vi "Example Graph.vi"() -> ()   [LabVIEW 2013]
uses:
  C:/tf/play/labview/Tinkerforge.dll
  Tinkerforge.dll
panel:
  in  "stop":bool
  out "graph":i32[](graph)
  in  "uid":string="amb"
  in  "port":i32=4223
  in  "host":string="localhost"
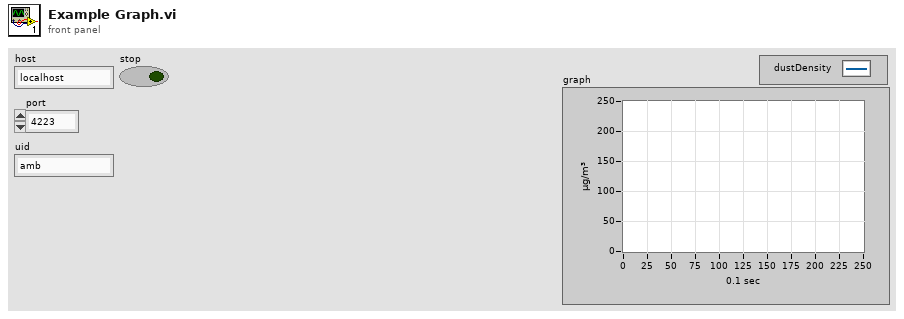
[diagram p1: front panel]
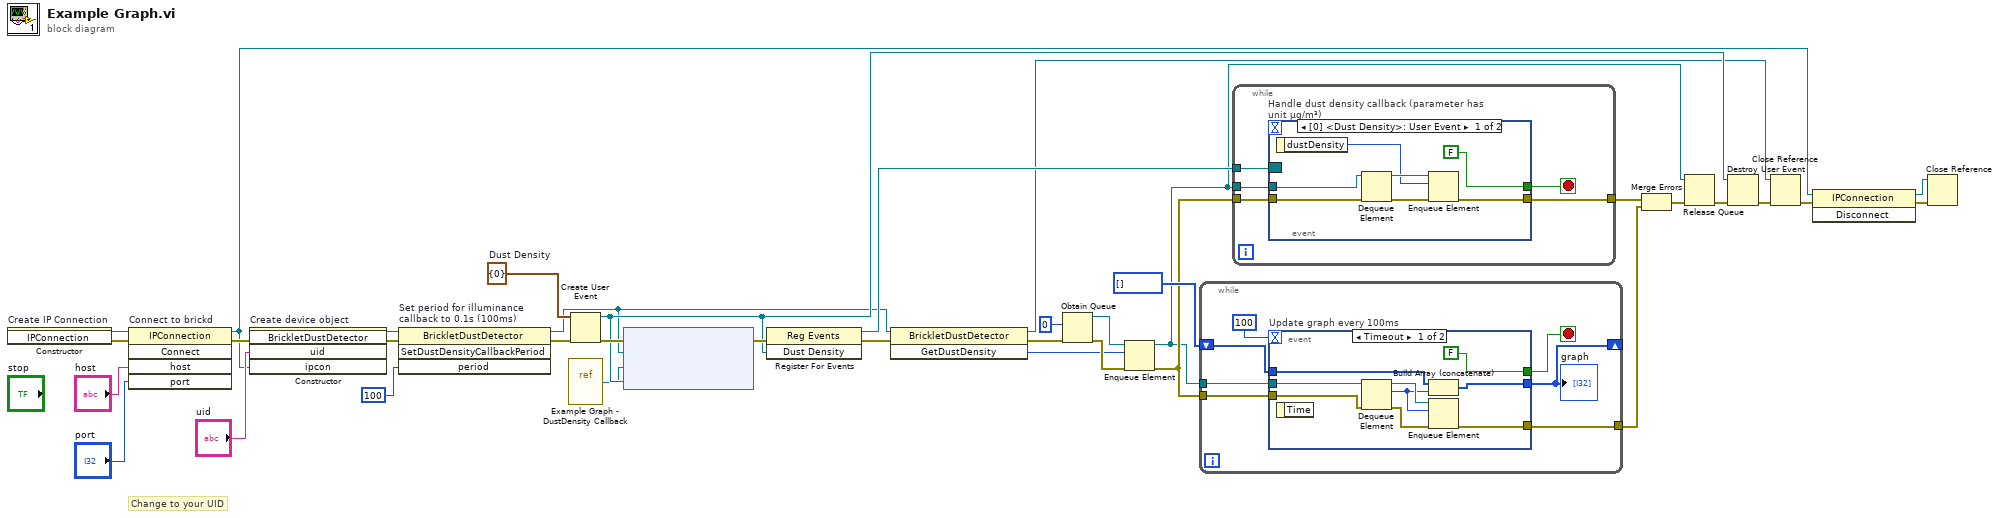
[diagram p0: block diagram]
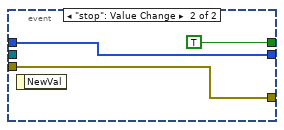
[diagram p2: hidden frame]
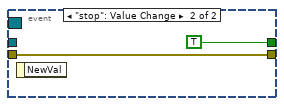
[diagram p3: hidden frame]
diagram:
  w22 = cluster{"dustDensity":i32} {"dustDensity"=0}  # Dust Density
  # "Change to your UID"
  n1 = constructor on="Create IP Connection" class="IPConnection"() -> (reference out=w36:refnum<k24>, error out=w7:errorcluster)  [unwired: 3 in, 1 out]
  n2 = invoke on="Connect to brickd" class="IPConnection" method="Connect"(reference=w36, error in=w7, "host"="host", "port"="port") -> (reference out=w29:refnum<k24>, error out=w32:errorcluster)  [unwired: 1 in, 3 out]
  n3 = constructor on="Create device object" class="BrickletDustDetector"(error in=w32, "uid"="uid", "ipcon"=w29) -> (reference out=w19:refnum<k24>, error out=w21:errorcluster)  [unwired: 2 in, 3 out]
  n4 = invoke on="Set period for illuminance\ncallback to 0.1s (100ms)" class="BrickletDustDetector" method="SetDustDensityCallbackPeriod"(reference=w19, error in=w21, "period"=i64 100) -> (reference out=w4:refnum<k24>, error out=w20:errorcluster)  [unwired: 1 in, 2 out]
  n5 = vi-ref "Example Graph - DustDensity Callback.vi"() -> ("vi reference"=w2:refnum<vi>)
  n6 = Create User Event(user event datatype=w22, error in=w20) -> (user event=w24:refnum<user-event>, error out=w27:errorcluster)
  n7 = node ("Register Event Callback")(w27, w4, w2, w24) -> (w26:errorcluster)  [unwired: 1 in, 1 out]
  n8 = register-events(error in=w26, w24) -> (reference out=w25:refnum<event-registration>, error out=w6:errorcluster)  [unwired: 1 in]
  n9 = invoke class="BrickletDustDetector" method="GetDustDensity"(reference=w4, error in=w6) -> (reference out=w3:refnum<k24>, error out=w5:errorcluster, "GetDustDensity"=w1:i32)  [unwired: 1 in]
  n10 = Obtain Queue(element data type=0, error in (no error)=w5) -> (queue out=w11:refnum<queue>, error out=w13:errorcluster)  [unwired: 3 in, 1 out]
  n11 = Enqueue Element(queue=w11, element=w1, error in (no error)=w13) -> (queue out=w8:refnum<queue>, error out=w12:errorcluster)  [unwired: 1 in, 1 out]
  n12 = while {
    tunnel: [w39] -> w17
    tunnel: w12 -> [w40]
    shift-right: [w41] -> _
    shift-left: i32[] [] -> [w42]
    tunnel: w8 -> [w38]
    stop <- w37 stop-if-true
    n13 = event "Update graph every 100ms" shown="[0] Timeout" {
      selector: _ -> [_ _]
      dyn-events: _ -> [_ _]
      timeout: 100 -> [_ _]
      tunnel: [w52 w54] -> w41
      tunnel: w42 -> [w45 w54]
      tunnel: w40 -> [w51 w53]
      tunnel: [w48 w53] -> w39
      tunnel: w38 -> [w50 _]
      tunnel: [FALSE TRUE] -> w37
      event Timeout {
        n14 = event-data() -> ()  [unwired: 1 in, 1 out]
        n15 = Dequeue Element(queue=w50, error in (no error)=w51) -> (queue out=w47:refnum<queue>, element=w46:i32, error out=w49:errorcluster)  [unwired: 1 in, 1 out]
        n16 = Build Array (concatenate)(w45, w46) -> (w52:i32[])
        n17 = Enqueue Element(queue=w47, element=w46, error in (no error)=w49) -> (error out=w48:errorcluster)  [unwired: 1 in, 2 out]
      }
      event "stop": Value Change {
        n18 = event-data() -> ()  [unwired: 1 in, 1 out]
      }
    }
    "graph" <- w41
  }
  n19 = while {
    tunnel: w25 -> [w60]
    tunnel: [w58] -> w16
    tunnel: w12 -> [w59]
    tunnel: w8 -> [w57]
    stop <- w56 stop-if-true
    n20 = event "Handle dust density callback (parameter has unit µg/m³)" shown="[0] <Dust Density>: User Event" {
      selector: w60 -> [_ _]
      dyn-events: _ -> [_ _]
      timeout: _ -> [_ _]
      tunnel: w59 -> [w67 w68]
      tunnel: [w65 w68] -> w58
      tunnel: w57 -> [w64 _]
      tunnel: [FALSE TRUE] -> w56
      event User Event {
        n21 = event-data() -> ("dustDensity"=w61:i32)  [unwired: 1 in]
        n22 = Dequeue Element(queue=w64, error in (no error)=w67) -> (queue out=w63:refnum<queue>, error out=w66:errorcluster)  [unwired: 1 in, 2 out]
        n23 = Enqueue Element(queue=w63, element=w61, error in (no error)=w66) -> (error out=w65:errorcluster)  [unwired: 1 in, 2 out]
      }
      event "stop": Value Change {
        n24 = event-data() -> ()  [unwired: 1 in, 1 out]
      }
    }
  }
  n25 = Merge Errors(w16, w17) -> (w10:errorcluster)
  n26 = Release Queue(queue=w8, error in (no error)=w10) -> (error out=w9:errorcluster)  [unwired: 1 in, 2 out]
  n27 = Destroy User Event(user event=w24, error in=w9) -> (error out=w23:errorcluster)
  n28 = Close Reference(reference=w3, error in (no error)=w23) -> (error out=w31:errorcluster)
  n29 = invoke class="IPConnection" method="Disconnect"(reference=w29, error in=w31) -> (reference out=w28:refnum<k24>, error out=w30:errorcluster)  [unwired: 1 in, 1 out]
  n30 = Close Reference(reference=w28, error in (no error)=w30) -> ()  [unwired: 1 out]
